vi "CppFunc.vi"(8 "Error In":errorcluster) -> (0 "Error Out":errorcluster)   [LabVIEW 2014]
uses:
  C_Library/C Basic Lib.lvlib
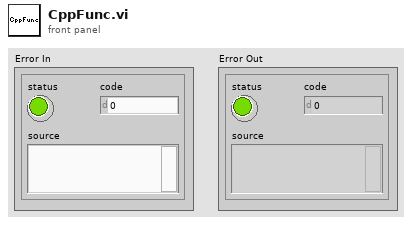
[diagram p1: front panel]
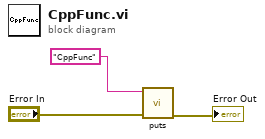
[diagram p0: block diagram]
diagram:
  n1 = call "puts.vi"("error in"="Error In", "String in"="CppFunc") -> ("error out"=→"Error Out":errorcluster)  [unwired: 9 in]
